vi "S2C_VLFT10_Proc_CreatePowerCurveLog.vi"(8 "Error In":errorcluster) -> (0 "Error Out":errorcluster)   [LabVIEW 2015]
uses:
  <vilib>/Utility/file.llb/Write Delimited Spreadsheet (string).vi
panel:
  out "FilePath":path
  out "FolderPath":path
  in  "Tester":string="1234"
  in  "SerialNumber":string="T3I70108DX"
  in  "FileDirectory":path=path "C:/Personal/Labview/S2C/Reports/VLFT10GEN/POWER CURVE"
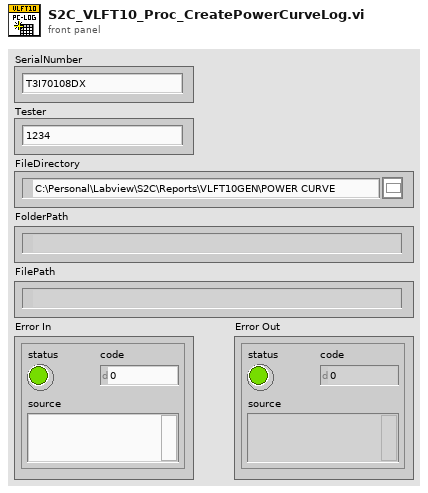
[diagram p1: front panel]
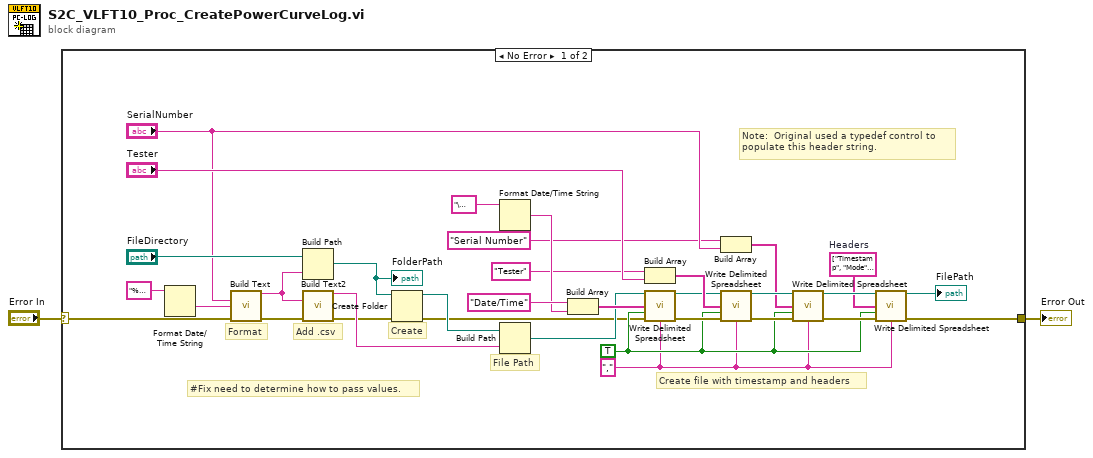
[diagram p0: block diagram]
diagram:
  n1 = case shown="No Error" "Error In" {
    selector: "Error In" -> [w32 w36]
    tunnel: [w33 w36] -> w1
    frame No Error {
      w5 = string[] ["Timestamp", "Mode", "Load", "Power", "Vin", "Iin", "Vrms", "Irms", "Pout", "Phase", "Vrms_MF_Sensor", "Irms_MF_Sensor", "Vrms_WB_Sensor", "Irms_WB_Sensor", "Vrms_Reg_Sensor", "Irms_Reg_Sensor", "V_Peak_Pos", "I_Peak_Pos", "VMagH1", "IMagH1", "ZMagH1", "VIPhaseH1", "IPhaseH1", "VMagH3", "IMagH3", "ZMagH3", "VIPhaseH3", "IPhaseH3", "VMagH5", "IMagH5", "ZMagH5", "VIPhaseH5", "IPhaseH5", "Control_Mode_HWC", "P_Real_MF_Sensor", "P_Real_WB_Sensor", "Z_Mag_Sensor", "Z_Phase_Sensor", "VMagH1_Sensor", "IMagH1_Sensor", "VIPhaseH1_Sensor", "VMagH3_Sensor", "IMagH3_Sensor", "VIPhaseH3_Sensor", "P_Accuracy_Percent", "P_Accuracy_Difference", "V_Accuracy_Percent", "V_Accuracy_Difference", "I_Accuracy_Percent", "I_Accuracy_Difference", "Z_Accuracy_Percent", "Z_Accuracy_Difference", "REM_Z", "P_HWC_Setpoint", "V_HWC_Setpoint", "I_HWC_Setpoint", "P_Real_Reg_Sensor", "Crest_Factor_V_Measured", "V_RMS_Redundant_Sensor", "I_RMS_Redundant_Sensor", "P_Real_Redundant_Sensor", "Z_Mag_Redundant_Sensor", "Z_Phase_Redundant_Sensor", "V_RMS_Sensor", "I_RMS_Sensor", "P_Real_Sensor", "Cal_Mode", "Sensor_Gain_Setting", "Crest_Factor_I_Measured", "V_Peak_Neg", "I_Peak_Neg", "Crest_Factor_I_Sensor", "Crest_Factor_V_Sensor", "I_Peak_Neg_Sensor", "I_Peak_Pos_Sensor", "V_Peak_Neg_Sensor", "V_Peak_Pos_Sensor", "Z_Imag_SF_Sensor", "Z_Real_SF_Sensor", "EnergyChannelID_Sensor", "Z_REM_Filtered_Sensor", "Mode_RF_Sensor", "Control_Mode_SWC", "Z_ABP_Filtered_Sensor", "Target_SWC_VIP", "VMagH5_Sensor", "IMagH5_Sensor", "VIPhaseH5_Sensor", "Power_LL", "Power_UL", "Voltage_LL", "Voltage_UL ", "Current_LL", "Current_UL", "Vpeak_UL", "HvpsVoltage", "HvpsCurrent", "Cphase", "Flags", "RfInverterFetTemperature", "CompSetPointP", "CompSetPointV", "Mode_Enum", "CammReceiptTimestampSeconds", "CammReceiptTimestampNanos", "NumSamples_Sensor", "RemFilteredZPhase", "CompLatchZ", "RemZPhase", "V_Reprate_Frequency_Measured", "I_Reprate_Frequency_Measured", "Z_Mag_Measured", "Z_Phase_Measured", "Impedance_LL", "Impedance_UL", "P_In", "Comment"]  # Headers
      w14 = TRUE
      w13 = "," ("delimiter (\\t)")
      # "#Fix need to determine how to pass values."
      # "Note:  Original used a typedef control to\npopulate this header string."
      # "Create file with timestamp and headers"
      # "File Path"
      # "Create"
      # "Add .csv"
      # "Format"
      n2 = Format Date/Time String(time format string (%c)="%Y%m%d%H%M%S") -> (date/time string=w12:string)  [unwired: 2 in]
      n3 = call "Build Text"("SN"="SerialNumber", "Time"=w12, "error in (no error)"=w32) -> ("Result"=w10:string, "error out"=w11:errorcluster)  [unwired: 11 in]
      n4 = Build Path(base path="FileDirectory", name or relative path=w10) -> (appended path=w3:path)
      "FolderPath" <- w3
      n5 = call "Build Text2"("File"=w10, "error in (no error)"=w11) -> ("Result"=w9:string, "error out"=w8:errorcluster)  [unwired: 12 in]
      n6 = Create Folder(path (use dialog)=w3, error in=w8) -> (created path=w7:path, error out=w6:errorcluster)  [unwired: 1 in, 1 out]
      n7 = Format Date/Time String(time format string (%c)="\"%A, %B %d, %Y %I:%M:%S%4u %p\"") -> (date/time string=w27:string)  [unwired: 2 in]
      n8 = Build Path(base path=w7, name or relative path=w9) -> (appended path=w25:path)
      n9 = Build Array("Date/Time", w27) -> (w26:string[])
      n10 = Build Array("Tester", "Tester") -> (w22:string[])
      n11 = call-poly <vilib>:"Write Delimited Spreadsheet.vi"("file path (dialog if empty)"=w25, "1D data"=w26, "append to file? (F)"=w14, "error in (no error)"=w6, "delimiter (\\t)"=w13) -> ("new file path (Not A Path if cancelled)"=w21:path, "error out"=w24:errorcluster)  [unwired: 9 in]
      n12 = Build Array("Serial Number", "SerialNumber") -> (w15:string[])
      n13 = call-poly <vilib>:"Write Delimited Spreadsheet.vi"("file path (dialog if empty)"=w21, "1D data"=w22, "append to file? (F)"=w14, "error in (no error)"=w24, "delimiter (\\t)"=w13) -> ("new file path (Not A Path if cancelled)"=w19:path, "error out"=w20:errorcluster)  [unwired: 9 in]
      n14 = call-poly <vilib>:"Write Delimited Spreadsheet.vi"("file path (dialog if empty)"=w19, "1D data"=w15, "append to file? (F)"=w14, "error in (no error)"=w20, "delimiter (\\t)"=w13) -> ("new file path (Not A Path if cancelled)"=w18:path, "error out"=w17:errorcluster)  [unwired: 9 in]
      n15 = call-poly <vilib>:"Write Delimited Spreadsheet.vi"("file path (dialog if empty)"=w18, "1D data"=w5, "append to file? (F)"=w14, "error in (no error)"=w17, "delimiter (\\t)"=w13) -> ("new file path (Not A Path if cancelled)"=→"FilePath":path, "error out"=w33:errorcluster)  [unwired: 9 in]
    }
    frame Error {
    }
  }
  "Error Out" <- w1
